vi "testUnflattenVelocityFromXML.vi"() -> ()   [LabVIEW 2012, in "UnitsAndXML.lvlib"]
uses:
  <userlib>/Common/UnitsAndXML/UnitsAndXML.lvlib
  <userlib>/Common/UnitsAndXML/FlattenItemWithUnitToXML/FlattenVelocityToXML/VelocityUnit.ctl
  <userlib>/Common/UnitsAndXML/UnflattenItemWithUnitFromXML/UnflattenVelocityFromXML/typeMethods/unflattenVelocityFromXML_Array.vi
  <userlib>/Common/UnitsAndXML/UnflattenItemWithUnitFromXML/UnflattenVelocityFromXML/typeMethods/unflattenVelocityFromXML_Scalar.vi
panel:
  out "error out":errorcluster
  out "velocity":dbl[unit][](array[numeric])
  out "velocity":dbl[unit]
  in  "velocityUnitInXML":T1
  in  "xmlStringArray":string="<velocity>15</velocity>\r\n<velocity>30</velocity>\r\n<velocity>45</velocity>\r\n<velocity>60</velocity>"
  in  "xmlStringScalar":string="<velocity>15</velocity>"
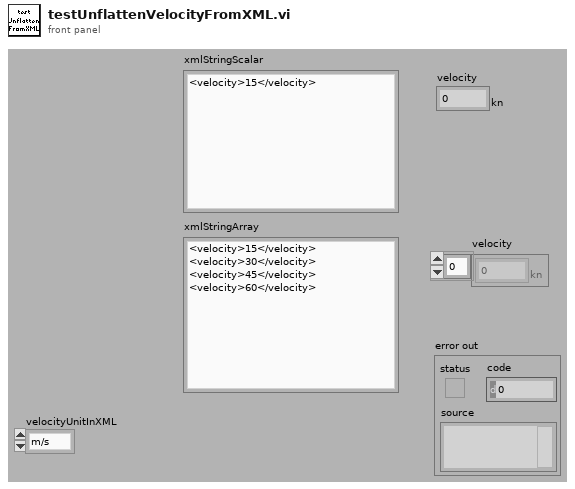
[diagram p1: front panel]
types:
  T1 = typedef "UnitsAndXML.lvlib/VelocityUnit.ctl" = enum16{"m/s", "km/s", "kn"}
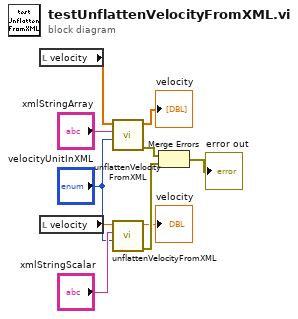
[diagram p0: block diagram]
diagram:
  n1 = local read "velocity"() -> (w3:dbl[unit][])
  n2 = local read "velocity"() -> (w10:dbl[unit])
  n3 = call-poly <userlib>:"unflattenVelocityFromXML.vi"("velocityUnitInXML"="velocityUnitInXML", "xmlString"="xmlStringArray", "velocityForType"=w3) -> ("error out"=w7:errorcluster, "velocity"=→"velocity":dbl[unit][])  [unwired: 7 in]
  n4 = call-poly <userlib>:"unflattenVelocityFromXML.vi"("velocityUnitInXML"="velocityUnitInXML", "xmlString"="xmlStringScalar", "velocityForType"=w10) -> ("error out"=w6:errorcluster, "velocity"=→"velocity":dbl[unit])  [unwired: 7 in]
  n5 = Merge Errors(w7, w6) -> (→"error out":errorcluster)
